vi "prepare.vi"(8 "error in (no error)":errorcluster, 11 "SweepDL090926Automation in":refnum<class "SweepDL090926Automation.lvclass">) -> (0 "error out":errorcluster, 3 "SweepDL090926Automation out":refnum<class "SweepDL090926Automation.lvclass">)   [LabVIEW 2010, in "SweepDL090926Automation.lvclass"]
uses:
  SweepDL090926Automation.lvclass
  GenericSweep/GenericSweep/GenericSweep.lvclass
  SweepDL090926Automation.lvclass/SweepDL090926Automation.ctl
  ImagingMode/GenericImagingMode/GenericImagingMode/GenericImagingMode.lvclass
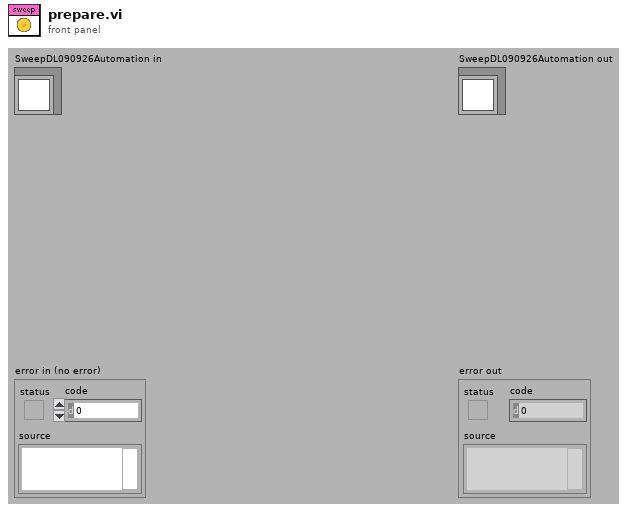
[diagram p1: front panel]
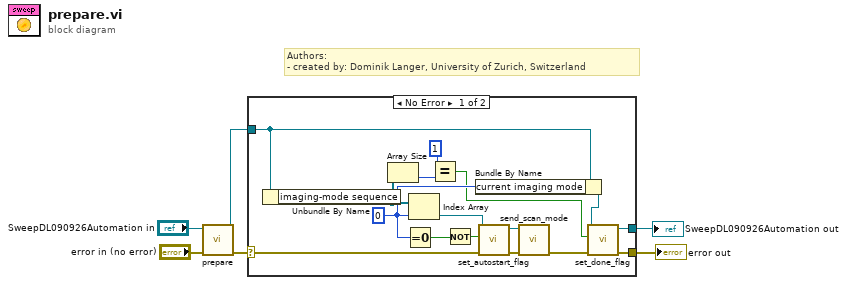
[diagram p0: block diagram]
diagram:
  # "Authors: \n- created by: Dominik Langer, University of Zurich, Switzerland"
  n1 = call-parent "prepare.vi"("error in (no error)"="error in (no error)", "GenericSweep in"="SweepDL090926Automation in") -> ("error out"=w4:errorcluster, "GenericSweep out"=w2:refnum<class "SweepDL090926Automation.lvclass">)  [unwired: 8 in]
  n2 = case shown="No Error" w4 {
    selector: w4 -> [w16 w23]
    tunnel: [w15 w23] -> w3
    tunnel: w2 -> [w13 w24]
    tunnel: [w14 w24] -> w1
    frame No Error {
      w12 = 0 ("t")
      n3 = Unbundle By Name(w13) -> ("imaging-mode sequence"=w10:refnum<class "GenericImagingMode.lvclass">[])
      n4 = Array Size(array=w10) -> (size(s)=w9:i32)
      n5 = Equal To 0?(x=w12) -> (x = 0?=w20:bool)
      n6 = Index Array(array=w10, index=w12) -> (element=w11:refnum<class "GenericImagingMode.lvclass">)
      n7 = Equal?(x=1, y=w9) -> (x = y?=w7:bool)
      n8 = Not(x=w20) -> (.not. x?=w19:bool)
      n9 = Bundle By Name(cluster=w13, "current imaging mode"=w12) -> (w17:refnum<class "SweepDL090926Automation.lvclass">)
      n10 = call-dynamic "set_autostart_flag.vi"("error in (no error)"=w16, "autostart?"=w19, "GenericScanMode in"=w11) -> ("error out"=w22:errorcluster, "GenericScanMode out"=w21:refnum<class "GenericImagingMode.lvclass">)  [unwired: 7 in]
      n11 = call-dynamic "send_scan_mode.vi"("error in (no error)"=w22, "GenericScanMode in"=w21) -> ("error out"=w18:errorcluster)  [unwired: 8 in, 1 out]
      n12 = call-dynamic "set_done_flag.vi"("error in (no error)"=w18, "done?"=w7, "GenericSweep in"=w17) -> ("error out"=w15:errorcluster, "GenericSweep out"=w14:refnum<class "SweepDL090926Automation.lvclass">)  [unwired: 7 in]
    }
    frame Error {
    }
  }
  "error out" <- w3
  "SweepDL090926Automation out" <- w1
